vi "Special_Processing.vi"(6 "cluster in":T1, 8 "error in (no error)":errorcluster, 9 "Terminal Map In":map{string, T3}(c390), 10 "Wires":T2[](array[typedef]), 11 "MultiDiagramStructure in":refnum<class "MultiDiagramStructure.lvclass">) -> (0 "error out":errorcluster, 1 "Terminal Map Out":map{string, T3}(c390), 2 "Wires out":T2[](array[typedef]), 3 "MultiDiagramStructure out":refnum<class "MultiDiagramStructure.lvclass">)   [LabVIEW 2025, in "MultiDiagramStructure.lvclass"]
uses:
  MultiDiagramStructure.lvclass
  Controls/wire.ctl
  Controls/Terminal.ctl
  Controls/bd.ctl
  Node.lvclass
  Structure.lvclass
  <vilib>/regexp/Match Regular Expression.xnode
  MultiDiagramStructure.lvclass/MultiDiagramStructure.ctl
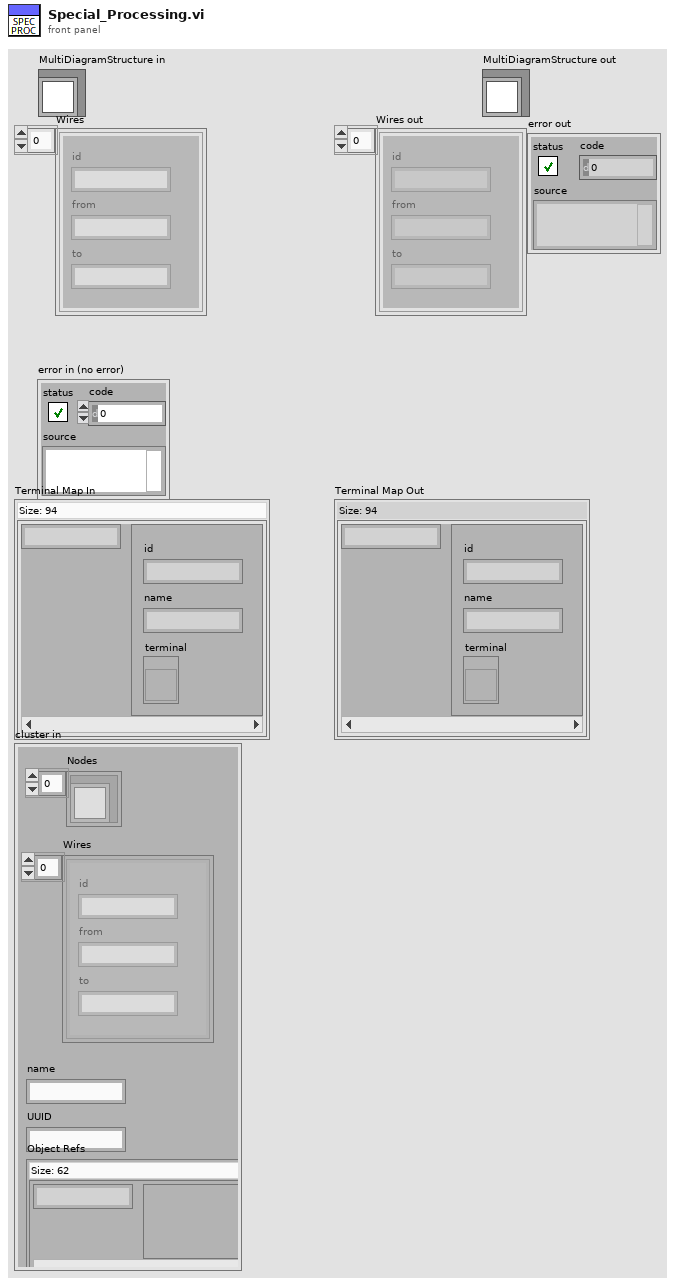
[diagram p1: front panel]
types:
  T1 = typedef "bd.ctl" = cluster{"Nodes":refnum<class "Node.lvclass">[], "Wires":T2[], "name":string, "UUID":string, "Object Refs":map{string, variant}}
  T2 = typedef "wire.ctl" = cluster{"id":string, "from":string, "to":string}
  T3 = typedef "Terminal.ctl" = cluster{"id":string, "name":string, "terminal":refnum<vi>}
  T4 = typedef "Tunnel.ctl" = cluster{"OuterUUID":T3, "InnerUUIDs":T3[]}
  T5 = typedef "Subdiagram.ctl" = cluster{"diagram":refnum<vi>, "selector":string, "uuid":string}
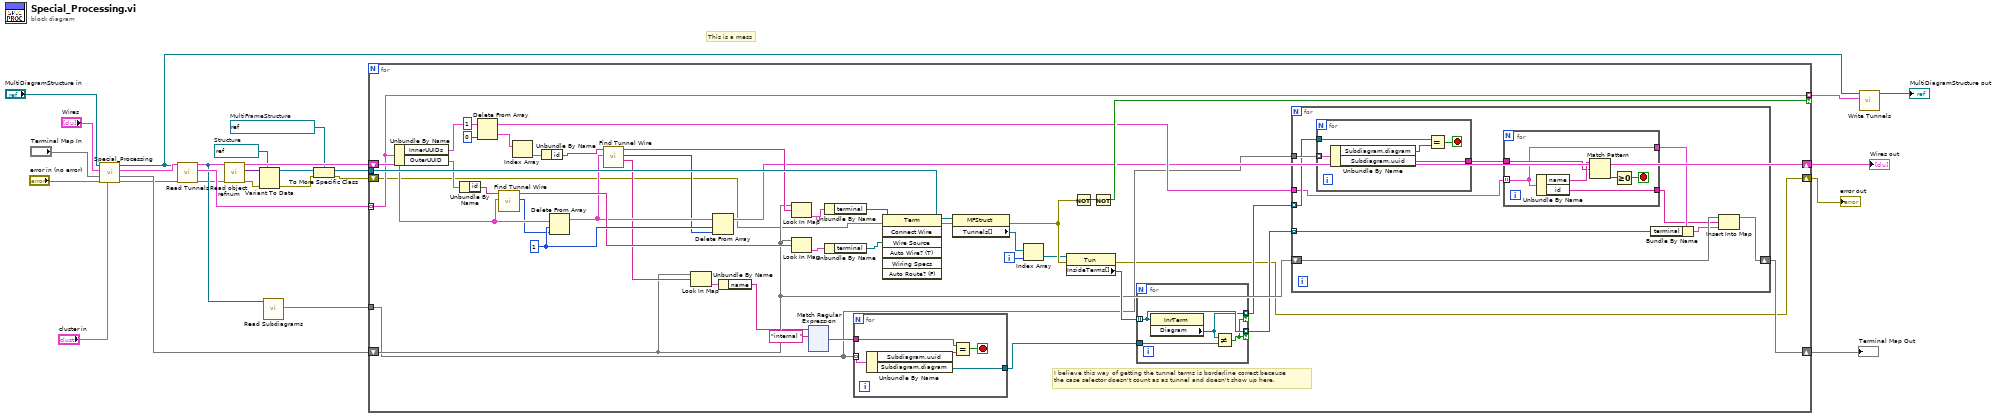
[diagram p0: block diagram]
diagram:
  w3 = refnum<vi> refnum  # MultiFrameStructure
  w16 = refnum<vi> refnum  # Structure
  # "This is a mess"
  n1 = call-parent "Special_Processing.vi"("cluster in"="cluster in", "error in (no error)"="error in (no error)", "Terminal Map In"="Terminal Map In", "Wires"="Wires", "Node in"="MultiDiagramStructure in") -> ("error out"=w8:errorcluster, "Terminal Map Out"=w22:map{string, T3}, "Wires out"=w23:T2[], "Node out"=w9:refnum<class "MultiDiagramStructure.lvclass">)  [unwired: 3 in]
  n2 = call-dynamic "Read Tunnels.vi"("error in (no error)"=w8, "Structure in"=w9) -> ("error out"=w7:errorcluster, "Tunnels"=w14:T4[], "Structure out"=w13:refnum<class "MultiDiagramStructure.lvclass">)  [unwired: 7 in]
  n3 = call-dynamic "Read object refnum.vi"("error in (no error)"=w7, "Node in"=w13) -> ("error out"=w6:errorcluster, "object refnum"=w17:variant)  [unwired: 7 in, 1 out]
  n4 = Variant To Data(error in=w6, type=w16, Variant=w17) -> (data=w15:refnum<vi>, error out=w2:errorcluster)
  n5 = call-dynamic "Read Subdiagrams.vi"("Structure in"=w13) -> ("Subdiagrams"=w12:map{u64, T5})  [unwired: 8 in, 2 out]
  n6 = To More Specific Class(target class=w3, reference=w15, error in=w2) -> (specific class reference=w4:refnum<vi>, error out=w1:errorcluster)
  n7 = for {
    shift-right: [w63] -> w20
    shift-left: w22 -> [w42]
    tunnel: w14 -> [w55] mode=indexing
    tunnel: w4 -> [w66]
    shift-right: [w35] -> w21
    shift-left: w23 -> [w61]
    tunnel: [w55] -> w10 mode=indexing if=w52
    tunnel: w12 -> [w30]
    shift-right: [w27] -> w5
    shift-left: w1 -> [w28]
    i -> [w65]
    w62 = 1 ("length")
    # "I believe this way of getting the tunnel terms is borderline correct because \nthe case selector doesn't count as as tunnel and doesn't show up here."
    n8 = Unbundle By Name(w55) -> ("InnerUUIDs"=w64:T3[], "OuterUUID"=w34:T3)
    n9 = Unbundle By Name(w34) -> ("id"=w33:string)
    n10 = Delete From Array(array=w64, length=1, index=0) -> (deleted portion=w45:T3[], array with subset deleted=w48:T3[])
    n11 = call "Find Tunnel Wire.vi"("Wires"=w61, "termUUID"=w33) -> ("Index"=w60:i32, "destination terminal"=w59:string)  [unwired: 7 in, 1 out]
    n12 = Index Array(array=w45) -> (element=w32:T3)  [unwired: 1 in]
    n13 = Unbundle By Name(w32) -> ("id"=w31:string)
    n14 = Delete From Array(array=w61, length=w62, index=w60) -> (array with subset deleted=w58:T2[])  [unwired: 1 out]
    n15 = call "Find Tunnel Wire.vi"("Wires"=w58, "termUUID"=w31) -> ("other_end"=w43:string, "Index"=w57:i32, "destination terminal"=w56:string)  [unwired: 7 in]
    n16 = Look In Map(map=w42, key=w43) -> (value=w41:T3)  [unwired: 1 in, 1 out]
    n17 = Delete From Array(array=w58, length=w62, index=w57) -> (array with subset deleted=w35:T2[])  [unwired: 1 out]
    n18 = Unbundle By Name(w41) -> ("name"=w40:string)
    n19 = Look In Map(map=w42, key=w56) -> (value=w69:T3)  [unwired: 1 in, 1 out]
    n20 = Look In Map(map=w42, key=w59) -> (value=w70:T3)  [unwired: 1 in, 1 out]
    n21 = xnode "Match Regular Expression"("input string"=w40, "regular expression"="internal ") -> ("after match"=w38:string)  [unwired: 4 in, 4 out]
    n22 = Unbundle By Name(w69) -> ("terminal"=w68:refnum<vi>)
    n23 = Unbundle By Name(w70) -> ("terminal"=w49:refnum<vi>)
    n24 = for {
      tunnel: w30 -> [w75] mode=indexing
      tunnel: w38 -> [w73]
      tunnel: [w71] -> w37
      stop <- w72 stop-if-true
      n25 = Unbundle By Name(w75) -> ("Subdiagram.uuid"=w74:string, "Subdiagram.diagram"=w71:refnum<vi>)
      n26 = Equal?(x=w73, y=w74) -> (x = y?=w72:bool)
    }
    n27 = invoke class="Term" method="Connect Wire"(reference=w68, error in=w28, "Wire Source"=w49) -> (error out=w67:errorcluster)  [unwired: 4 in, 6 out]
    n28 = property class="MFStruct"(reference=w66, error in=w67) -> (error out=w54:errorcluster, "Tunnels[]"=w50:refnum<vi>[])  [unwired: 1 out]
    n29 = Index Array(array=w50, index=w65) -> (element=w51:refnum<vi>)
    n30 = property class="Tun"(reference=w51, error in=w54) -> (error out=w27:errorcluster, "InsideTerms[]"=w44:refnum<vi>[])  [unwired: 1 out]
    n31 = Not(x=w54) -> (.not. x?=w53:bool)
    n32 = Not(x=w53) -> (.not. x?=w52:bool)
    n33 = for {
      tunnel: w44 -> [w195] mode=indexing
      tunnel: [w195] -> w36 mode=indexing if=w193
      tunnel: w37 -> [w196]
      tunnel: [w194] -> w29 mode=indexing if=w193
      n34 = property class="InrTerm"(reference=w195) -> ("Diagram"=w194:refnum<vi>)  [unwired: 1 in, 2 out]
      n35 = Not Equal?(x=w194, y=w196) -> (x != y?=w193:bool)
    }
    n36 = for {
      tunnel: w48 -> [w200]
      tunnel: w36 -> [w206] mode=indexing
      shift-right: [w205] -> w63
      shift-left: w42 -> [w204]
      tunnel: w30 -> [w203]
      tunnel: w29 -> [w202] mode=indexing
      n37 = for {
        tunnel: w203 -> [w217] mode=indexing
        tunnel: w202 -> [w214]
        tunnel: [w213] -> w201
        stop <- w216 stop-if-true
        n38 = Unbundle By Name(w217) -> ("Subdiagram.diagram"=w215:refnum<vi>, "Subdiagram.uuid"=w213:string)
        n39 = Equal?(x=w214, y=w215) -> (x = y?=w216:bool)
      }
      n40 = for {
        tunnel: w201 -> [w211]
        tunnel: w200 -> [w208] mode=indexing
        tunnel: [w208] -> w199
        tunnel: [w207] -> w197
        stop <- w209 stop-if-true
        n41 = Unbundle By Name(w208) -> ("name"=w212:string, "id"=w207:string)
        n42 = Match Pattern(string=w212, regular expression=w211) -> (offset past match=w210:i32)  [unwired: 1 in, 3 out]
        n43 = Greater Or Equal To 0?(x=w210) -> (x >= 0?=w209:bool)
      }
      n44 = Bundle By Name(cluster=w199, "terminal"=w206) -> (w198:T3)
      n45 = Insert Into Map(map in=w204, key=w197, value=w198) -> (map out=w205:map{string, T3})  [unwired: 2 out]
    }
  }
  "Wires out" <- w21
  "Terminal Map Out" <- w20
  "error out" <- w5
  n46 = call-dynamic "Write Tunnels.vi"("Tunnels"=w10, "Structure in"=w9) -> ("Structure out"=→"MultiDiagramStructure out":refnum<class "MultiDiagramStructure.lvclass">)  [unwired: 8 in, 1 out]
